vi "Scale by 2.vi"(0 "input data":T1[](array[typedef])=[{"I"=0.0, "Q"=0.0, "overflow"=FALSE}, {"I"=0.0, "Q"=0.0, "overflow"=FALSE}, {"I"=0.0, "Q"=0.0, "overflow"=FALSE}, {"I"=0.0, "Q"=0.0, "overflow"=FALSE}], 9 "input valid":bool, 11 "acq in":refnum<class "niUSRP Rx DSP v2 FPGA.lvclass">) -> (4 "output data":T1[](array[typedef]), 10 "output valid":bool, 15 "acq out":refnum<class "niUSRP Rx DSP v2 FPGA.lvclass">)   [LabVIEW 2025, in "niUSRP Rx DSP v2 FPGA.lvclass"]
doc: "Rescales the 'input data' signal level to compensate for the halved power artifact of digital downconversion."
uses:
  niUSRP Rx DSP v2 FPGA.lvclass
  <instrlib>/_niInstr/DSP/v1/Shared/Public/IQ Data.ctl
  <vilib>/rvi/DataTransferAndStorage/Container/XNode/niFpgaContainer.xnode
  <instrlib>/_niInstr/Basic Elements/v1/FPGA/niInstr Basic Elements v1 FPGA.lvlib
  <instrlib>/_niInstr/DSP/v1/Shared/niInstr DSP v1 Shared.lvlib
  <instrlib>/_niInstr/Basic Elements/v1/FPGA/Public/Max Fanout.ctl
  <vilib>/rvi/DataTransferAndStorage/Register/Emulation/niFpgaRegisterEmulationRefIn.vi
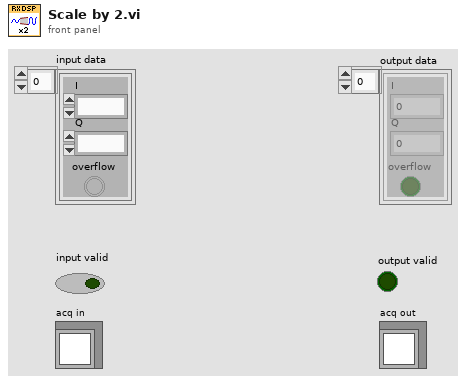
[diagram p1: front panel]
types:
  T1 = typedef "niInstr DSP v1 Shared.lvlib/IQ Data.ctl" = cluster{"I":fxp<+/-,18,1>, "Q":fxp<+/-,18,1>, "overflow":bool}
  T2 = typedef "niInstr Basic Elements v1 FPGA.lvlib/Max Fanout.ctl" = enum16{"4", "8", "16", "32"}
  T3 = typedef "niUSRP Rx DSP v2 FPGA.lvclass/DSP Shared Regs.ctl" = cluster{"rfsa.abort":refnum<k21>, "reset":refnum<k21>, "reset.done":refnum<k21>, "RxDspEnabled":refnum<k21>}
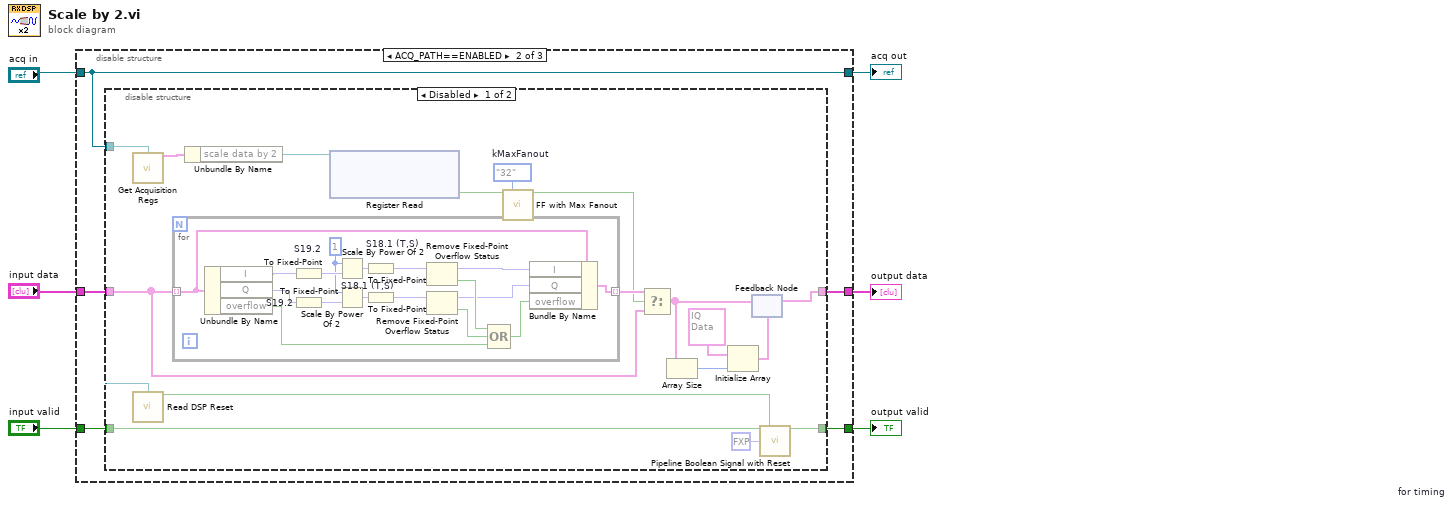
[diagram p0: block diagram]
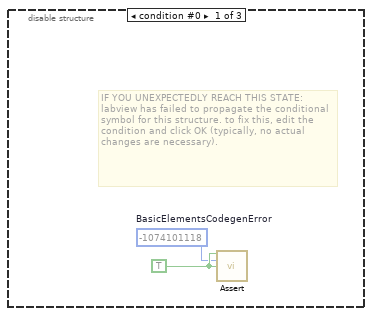
[diagram p2: hidden frame]
diagram:
  n1 = disable-structure shown="ACQ_PATH==ENABLED" {
    disable-tunnel: "input data" -> [_ w13 w52]
    disable-tunnel: [_ w10 w52] -> w5
    disable-tunnel: "input valid" -> [_ w11 w50]
    disable-tunnel: "acq in" -> [_ w9 w51]
    disable-tunnel: [_ w12 w50] -> w2
    disable-tunnel: [_ w9 w51] -> w1
    frame condition #0 {
      w8 = TRUE ("assert")
      w7 = -1074101118  # BasicElementsCodegenError
      # "IF YOU UNEXPECTEDLY REACH THIS STATE:\nlabview has failed to propagate the conditional symbol for this structure. to fix this, edit the condition and click OK (typically, no actual changes are necessary)."
      n2 = call <instrlib>:"Assert.vi"("assert"=w8, "error code"=w7, "enable show error"=w8) -> ()  [unwired: 13 in]
    }
    frame condition #1 (active) {
      n3 = disable-structure shown="Disabled" {
        disable-tunnel: w13 -> [w28 w49]
        disable-tunnel: [w26 w48] -> w12
        disable-tunnel: w11 -> [w25 w48]
        disable-tunnel: [w24 w49] -> w10
        disable-tunnel: w9 -> [w14 _]
        frame Disabled {
          w17 = Max_Fanout."32"  # kMaxFanout
          n4 = call-dynamic "Get Acquisition Regs.vi"("acq"=w14) -> ("dsp"=w15:T3)  [unwired: 14 in]
          n5 = call-dynamic "Read DSP Reset.vi"("acq"=w14) -> ("dsp reset"=w27:bool)  [unwired: 14 in]
          n6 = for {
            tunnel: w28 -> [w31] mode=indexing
            tunnel: [w32] -> w29 mode=indexing
            w36 = i16 1 ("n")
            n7 = Unbundle By Name(w31) -> ("I"=w39:fxp<+/-,18,1>, "Q"=w38:fxp<+/-,18,1>, "overflow"=w37:bool)
            n8 = To Fixed-Point "S19.2"(number=w39) -> (fixed-point=w40:fxp<+/-,19,2>)  [unwired: 1 in]
            n9 = To Fixed-Point "S19.2"(number=w38) -> (fixed-point=w41:fxp<+/-,19,2>)  [unwired: 1 in]
            n10 = Scale By Power Of 2(n=w36, x=w40) -> (x*2^n=w42:fxp<+/-,19,2>)
            n11 = Scale By Power Of 2(n=w36, x=w41) -> (x*2^n=w43:fxp<+/-,19,2>)
            n12 = To Fixed-Point "S18.1 (T,S)"(number=w42) -> (fixed-point=w44:fxp<+/-,18,1>)  [unwired: 1 in]
            n13 = To Fixed-Point "S18.1 (T,S)"(number=w43) -> (fixed-point=w45:fxp<+/-,18,1>)  [unwired: 1 in]
            n14 = Remove Fixed-Point Overflow Status(3:w44) -> (0:w46:bool, 1:w35:fxp<+/-,18,1>)
            n15 = Remove Fixed-Point Overflow Status(3:w45) -> (0:w47:bool, 1:w34:fxp<+/-,18,1>)
            n16 = Compound Arithmetic op=OR(w46, w47, w37) -> (w33:bool)
            n17 = Bundle By Name(cluster=w31, "I"=w35, "Q"=w34, "overflow"=w33) -> (w32:T1)
          }
          n18 = Unbundle By Name(w15) -> ("scale data by 2"=w30:refnum<k21>)
          n19 = xnode ("Register Read")("Register In"=w30) -> ("Data"=w18:bool)  [unwired: 1 out]
          n20 = call <instrlib>:"FF with Max Fanout.vi"("cDataIn"=w18, "kMaxFanout"=w17) -> ("cDataOut"=w16:bool)  [unwired: 13 in]
          n21 = Select(t=w29, s=w16, f=w28) -> (s? t:f=w20:T1[])
          n22 = Array Size(array=w20) -> (size(s)=w22:i32)
          n23 = Initialize Array(T1 {"I"=0.0, "Q"=0.0, "overflow"=FALSE} ("data"), w22) -> (w21:T1[])
          n24 = feedback #1 "for timing"(w21) -> (w24:T1[])
          n25 = feedback-in #1(w20) -> ()
          n26 = call <instrlib>:"Pipeline Boolean Signal with Reset.vi"("input signal"=w25, "reset"=w27, "delay"=fxp<+,6,6> 1.0) -> ("output signal"=w26:bool)  [unwired: 12 in]
        }
        frame Enabled {
        }
      }
    }
    frame condition #2 {
    }
  }
  "output data" <- w5
  "output valid" <- w2
  "acq out" <- w1
